vi "Status Append.vi"(0 "New Status Out":string, 3 "New Status In":string, 4 "Status Log In":string) -> (1 "Status Log Out":string, 2 "Time Stamped Status String":string)   [LabVIEW 2019]
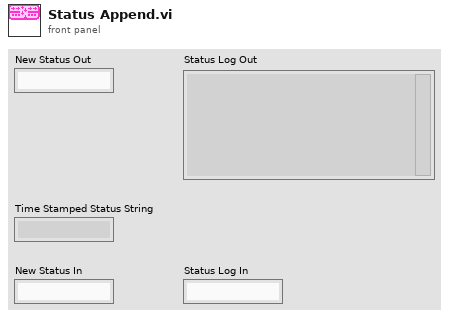
[diagram p1: front panel]
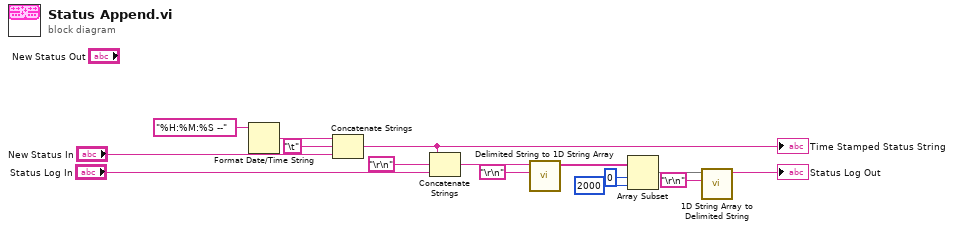
[diagram p0: block diagram]
diagram:
  n1 = Format Date/Time String(time format string (%c)="%H:%M:%S --") -> (date/time string=w14:string)  [unwired: 2 in]
  n2 = Concatenate Strings(w14, "\t", "New Status In") -> (w1:string)
  "Time Stamped Status String" <- w1
  n3 = Concatenate Strings(w1, "\r\n", "Status Log In") -> (w7:string)
  n4 = call <vilib>:"Delimited String to 1D String Array.vi"("delimiter"="\r\n", "delimited string"=w7) -> ("string array"=w12:string[])  [unwired: 9 in]
  n5 = Array Subset(array=w12, index=0, length=2000) -> (w9:string[])
  n6 = call <vilib>:"1D String Array to Delimited String.vi"("delimiter"="\r\n", "string array"=w9) -> ("delimited string"=→"Status Log Out":string)  [unwired: 9 in]
